vi "LinxUartRead.vi"(8 "Error In":errorcluster, 9 "Num Bytes":u8, 10 "Uart Channel":u8, 11 "LINX Resource":T1) -> (0 "Error Out":errorcluster, 1 "Num Bytes Read":u8, 2 "Data":u8[](array[numeric]), 3 "LINX Resource":T1)   [LabVIEW 2020, in "LMH-LINX.lvlib" / "Local IO.lvlib"]
uses:
  Local IO.lvlib
  Type Defs/LINX Ref.ctl
  Type Defs/Platform.ctl
  Device/Type Defs/LINX Device Config.ctl
  Type Defs/Interface.ctl
  Device/Type Defs/TCP Config.ctl
  Device/Type Defs/Channels.ctl
  Type Defs/Error Type.ctl
  LMH-LINX.lvlib
  Type Defs/Channel FGV States.ctl
  E:/lv2019/dist/vi.lib/MakerHub/LINX/Resources/liblinxdevice.dll
  Device/Device.lvlib
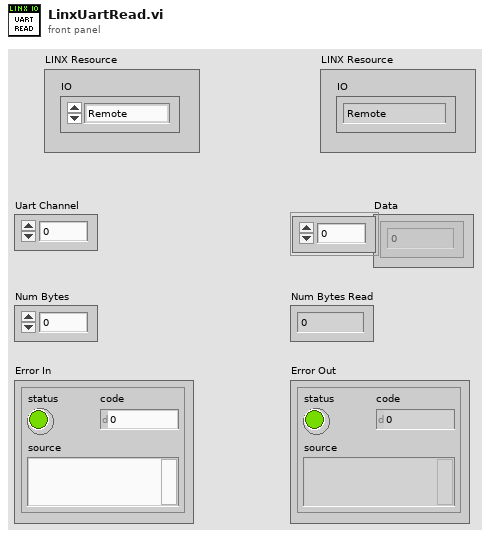
[diagram p1: front panel]
types:
  T1 = typedef "LMH-LINX.lvlib/LINX Ref.ctl" = cluster{"IO":T2, "LINX Device Config":T3}
  T2 = typedef "LMH-LINX.lvlib/Platform.ctl" = enum16{"Remote", "Local"}
  T3 = typedef "Device.lvlib/LINX Device Config.ctl" = cluster{"Interface":T4, "COM Port":refnum<visa-resource-name>, "TCP Configuration":T5, "Device Family":u8, "Device ID":u8, "Device Name":string, "TCP Ref":refnum<k5>, "Local Refnum":u64, "Channels":T6}
  T4 = typedef "LMH-LINX.lvlib/Interface.ctl" = enum16{"Serial", "TCP"}
  T5 = typedef "Device.lvlib/TCP Config.ctl" = cluster{"IP Address":string, "Port":u16}
  T6 = typedef "LMH-LINX.lvlib/Channels.ctl" = cluster{"DI":u8[], "DO":u8[], "AI":u8[], "AO":u8[], "PWM":u8[], "QE":u8[], "UART":u8[], "I2C 2":u8[], "SPI":u8[], "CAN":u8[], "Servo":u8[], "AI Ref (V)":dbl, "AI Resolution (Bits)":u8, "AO Ref (V)":dbl, "AO Resolution (Bits)":u8}
  T7 = typedef "LMH-LINX.lvlib/Error Type.ctl" = enum16{"Unknown", "Timeout", "Corrupt Return Packet", "Unable To Connect", "Command Not Supported", "Channel DNE", "Invalid COM Config", "Firmware Version Mismatch", "myRIO Support", "CMD Specific Error", "Local IO Not Supported"}
  T8 = typedef "LMH-LINX.lvlib/Channel FGV States.ctl" = enum16{"Initialize", "Get", "Set"}
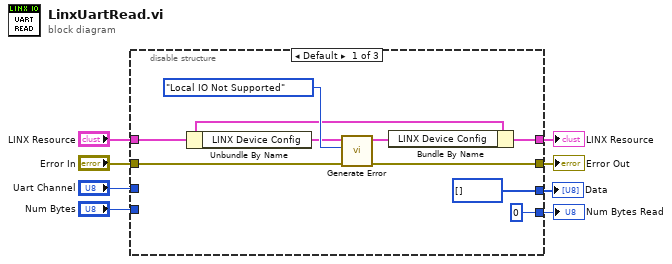
[diagram p0: block diagram]
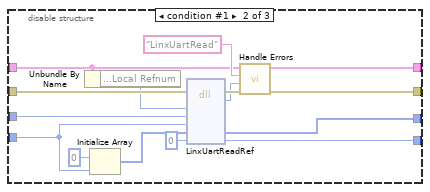
[diagram p2: hidden frame]
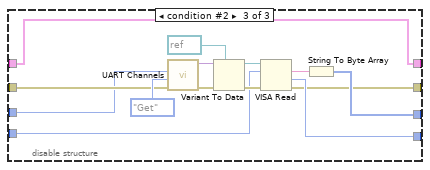
[diagram p3: hidden frame]
diagram:
  n1 = disable-structure shown="Default" {
    disable-tunnel: [w11 w30 w38] -> w7
    disable-tunnel: "LINX Resource" -> [w13 w19 w38]
    disable-tunnel: "Error In" -> [w16 w32 w39]
    disable-tunnel: [w15 w28 w35] -> w8
    disable-tunnel: "Uart Channel" -> [_ w31 w34]
    disable-tunnel: "Num Bytes" -> [_ w25 w33]
    disable-tunnel: [u8 0 ("Baud Rate") w21 w36] -> w2
    disable-tunnel: [u8[] [] ("Data") w20 w37] -> w1
    frame condition #0 (active) {
      n2 = Unbundle By Name(w13) -> ("LINX Device Config"=w14:T3)
      n3 = call "Generate Error.vi"("Error In"=w16, "Error Type"=Error_Type."Local IO Not Supported", "LINX Device Config"=w14) -> ("Error Out"=w15:errorcluster, "Dup LINX Device Config"=w12:T3)  [unwired: 7 in]
      n4 = Bundle By Name(cluster=w13, "LINX Device Config"=w12) -> (w11:T1)
    }
    frame condition #1 {
      n5 = Unbundle By Name(w19) -> ("LINX Device Config.Local Refnum"=w18:u64)
      n6 = Initialize Array(u8 0 ("element"), w25) -> (w23:u8[])
      n7 = dll-call lib="E:/lv2019/dist/vi.lib/MakerHub/LINX/Resources/liblinxdevice.*" fn="LinxUartReadRef"(error in=w32, "refnum"=w18, "channel"=w31, "numBytes"=w25, "recBuffer"=w23, "numBytesRead"=u8 0) -> (error out=w29:errorcluster, "status"=w26:i32, "recBuffer"=w20:u8[], "numBytesRead"=w21:u8)  [unwired: 5 in, 1 out]
      n8 = call "Handle Errors.vi"("Error In"=w29, "LinxStatus"=w26, "Function Name"="LinxUartRead", "LINX Resource"=w19) -> ("Error Out"=w28:errorcluster, "LINX Resource"=w30:T1)  [unwired: 6 in]
    }
    frame condition #2 {
      n9 = call "UART Channels.vi"("Error In"=w39, "Channel State"=Channel_FGV_States."Get", "Channel Number"=w34) -> ("Error Out"=w40:errorcluster, "UART Channel"=w41:variant)  [unwired: 7 in]
      n10 = Variant To Data(error in=w40, type=refnum<visa-resource-name> refnum ("reference"), Variant=w41) -> (data=w44:refnum<visa-resource-name>, error out=w45:errorcluster)
      n11 = VISA Read(VISA resource name=w44, byte count=w33, error in (no error)=w45) -> (read buffer=w46:string, return count=w36:u32, error out=w35:errorcluster)  [unwired: 1 out]
      n12 = String To Byte Array(string=w46) -> (unsigned byte array=w37:u8[])
    }
  }
  "LINX Resource" <- w7
  "Num Bytes Read" <- w2
  "Error Out" <- w8
  "Data" <- w1
